vi "Geometric Mean.vi"(10 "Array - Numeric":dbl[](array[numeric])) -> (2 "Geometric Mean":dbl)   [LabVIEW 2014]
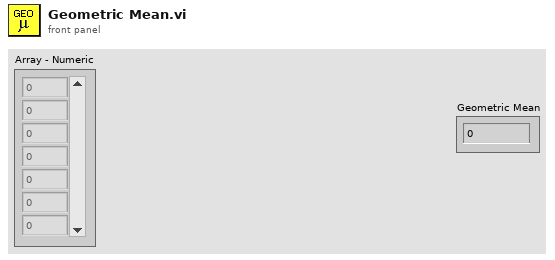
[diagram p1: front panel]
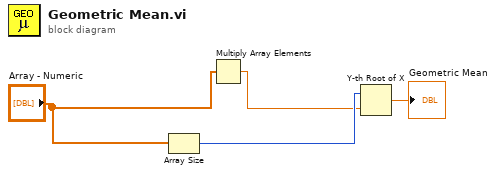
[diagram p0: block diagram]
diagram:
  n1 = Array Size(array="Array - Numeric") -> (size(s)=w3:i32)
  n2 = Multiply Array Elements(1:"Array - Numeric") -> (0:w2:dbl)
  n3 = Y-th Root of X(1:w2, 2:w3) -> (0:→"Geometric Mean":dbl)
